vi "Pointer.Read (1D Boolean).vi"(8 "error in (no error)":errorcluster, 10 "count":i32, 11 "pointer in":u64) -> (0 "error out":errorcluster, 2 "values":bool[](array[boolean]), 3 "pointer out":u64)   [LabVIEW 2016, in "VeriStand Data.lvlib"]
doc: "Reads a number of values, specified by <B>count</B>, from the provided <B>pointer</B>."
uses:
  VeriStand Data.lvlib
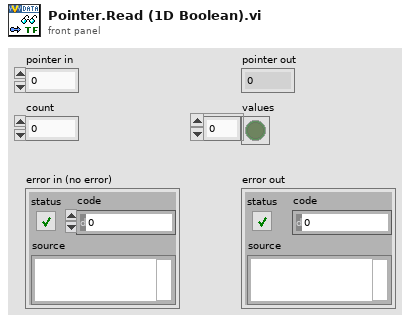
[diagram p1: front panel]
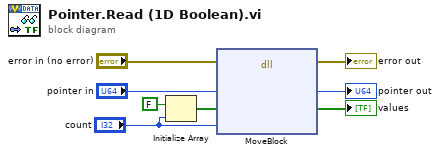
[diagram p0: block diagram]
diagram:
  n1 = Initialize Array(FALSE, "count") -> (w2:bool[])
  n2 = dll-call lib="LabVIEW" fn="MoveBlock"(error in="error in (no error)", "ps"="pointer in", "pd"=w2, "size"="count") -> (error out=→"error out":errorcluster, "ps"=→"pointer out":u64, "pd"=→"values":bool[])  [unwired: 4 in, 1 out]
